vi "Answer Received.vi"(8 "error in (no error)":errorcluster, 9 "Correct?":bool, 10 "Contestant":i32, 11 "Controller in":refnum<class "Controller.lvclass">) -> (0 "error out":errorcluster, 3 "Controller out":refnum<class "Controller.lvclass">)   [LabVIEW 2024, in "Controller.lvlib" / "Controller.lvclass"]
uses:
  Controller.lvclass
  C:/Program Files/National Instruments/LabVIEW 2024/vi.lib/ActorFramework/Actor/Actor.lvclass
  Controller.lvclass/Controller.ctl
  <vilib>/ActorFramework/Message Enqueuer/Message Enqueuer.lvclass/Message Enqueuer.ctl
  Contestant/Contestant Messages/Decrement Score Msg/Decrement Score Msg.lvclass/Decrement Score Msg.ctl
  <vilib>/ActorFramework/Actor/Actor.lvclass/Actor.ctl
  Controller Messages/Update Player Who Answered Correctly Last Msg/Update Player Who Answered Correctly Last Msg.lvclass/Update Player Who Answered Correctly Last Msg.ctl
  Contestant/Contestant Messages/Increment Score Msg/Increment Score Msg.lvclass/Increment Score Msg.ctl
  <vilib>/ActorFramework/Message Enqueuer/Enqueue.vi
  <vilib>/ActorFramework/Message Enqueuer/Init from Existing Queue.vi
  Timer/Timer Messages/Stop Timer Msg/Stop Timer Msg.lvclass
  C:/Program Files/National Instruments/LabVIEW 2024/vi.lib/ActorFramework/Message/Message.lvclass
  Contestant/Contestant Messages/Decrement Score Msg/Decrement Score Msg.lvclass
  Contestant/Contestant Messages/Light to Red Msg/Light to Red Msg.lvclass
  Controller Messages/Update Player Who Answered Correctly Last Msg/Update Player Who Answered Correctly Last Msg.lvclass
  Contestant/Contestant Messages/Increment Score Msg/Increment Score Msg.lvclass
  <vilib>/ActorFramework/Message Priority Queue/Priority Enqueue.vi
  <vilib>/ActorFramework/Message Enqueuer/Message Enqueuer.lvclass
  <vilib>/ActorFramework/Actor/Actor.lvclass
  C:/Users/ekerry/Documents/challenge-of-champions/Controller/Controller/Controller.lvclass
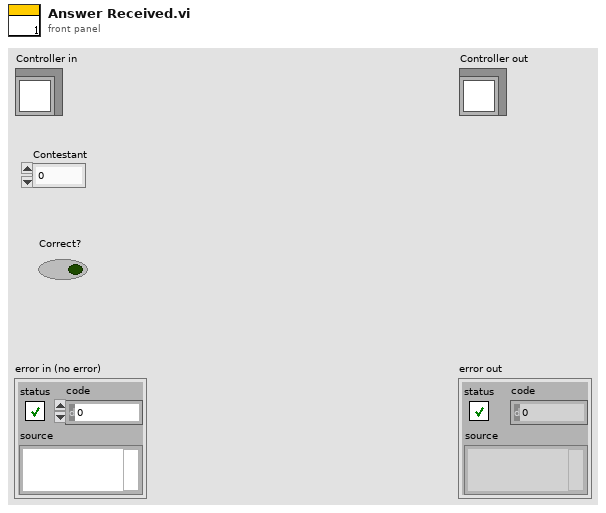
[diagram p1: front panel]
types:
  T1 = map{i32, refnum<class "Message Enqueuer.lvclass">}
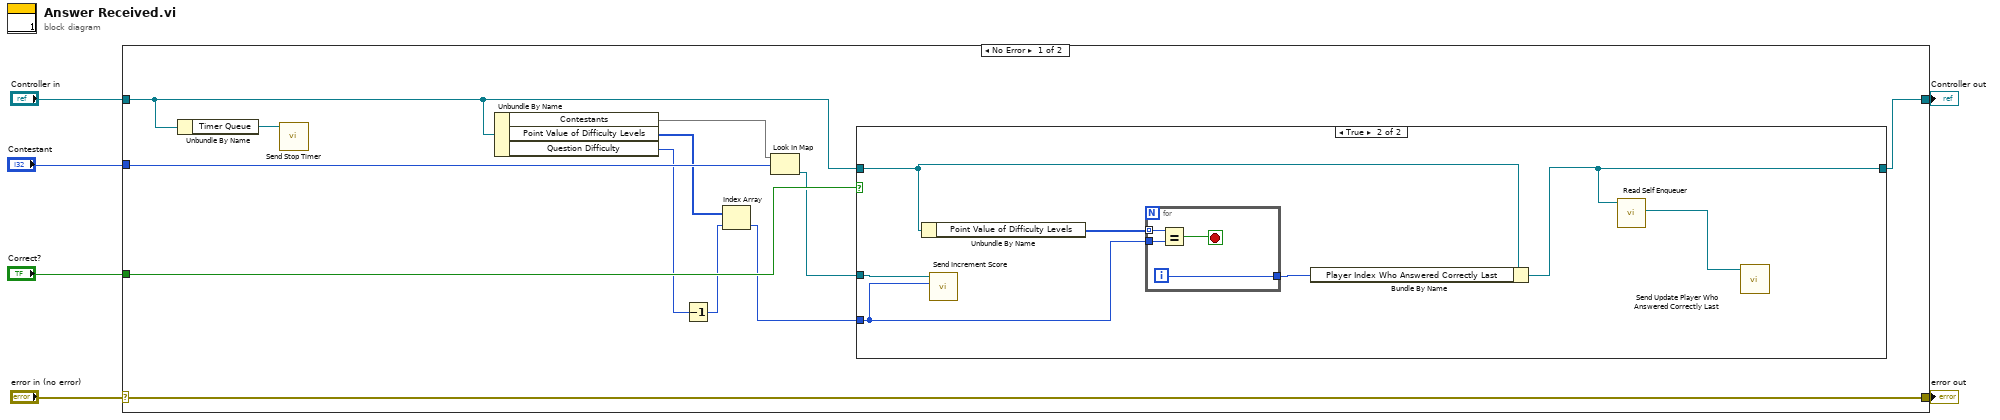
[diagram p0: block diagram]
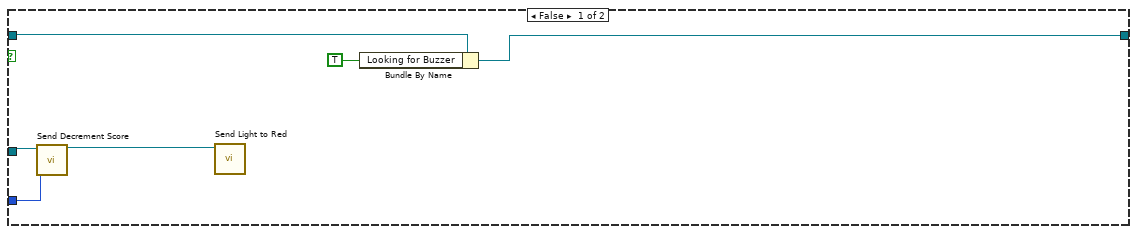
[diagram p2: hidden frame]
diagram:
  n1 = case shown="No Error" "error in (no error)" {
    selector: "error in (no error)" -> [w18 w37]
    tunnel: [w18 w37] -> w5
    tunnel: [w9 w36] -> w3
    tunnel: "Controller in" -> [w8 w36]
    tunnel: "Contestant" -> [w16 _]
    tunnel: "Correct?" -> [w15 _]
    frame No Error {
      n2 = Unbundle By Name(w8) -> ("Timer Queue"=w7:refnum<class "Message Enqueuer.lvclass">)
      n3 = call "Send Stop Timer.vi"("Message Enqueuer"=w7) -> ()  [unwired: 9 in, 2 out]
      n4 = Unbundle By Name(w8) -> ("Contestants"=w17:T1, "Point Value of Difficulty Levels"=w13:i32[], "Question Difficulty"=w11:i32)
      n5 = Decrement(x=w11) -> (x-1=w10:i32)
      n6 = Index Array(array=w13, index=w10) -> (element=w12:i32)
      n7 = Look In Map(map=w17, key=w16) -> (value=w14:refnum<class "Message Enqueuer.lvclass">)  [unwired: 1 in, 1 out]
      n8 = case shown="True" w15 {
        tunnel: w14 -> [w21 w31]
        tunnel: w12 -> [w20 w28]
        tunnel: w8 -> [w24 w27]
        tunnel: [w23 w26] -> w9
        frame False {
          n9 = call "Send Decrement Score.vi"("Points Lost"=w20, "Message Enqueuer"=w21) -> ("Message Enqueuer out"=w19:refnum<class "Message Enqueuer.lvclass">)  [unwired: 8 in, 1 out]
          n10 = call "Send Light to Red.vi"("Message Enqueuer"=w19) -> ()  [unwired: 9 in, 2 out]
          n11 = Bundle By Name(cluster=w24, "Looking for Buzzer"=TRUE) -> (w23:refnum<class "Controller.lvclass">)
        }
        frame True {
          n12 = Unbundle By Name(w27) -> ("Point Value of Difficulty Levels"=w29:i32[])
          n13 = call "Send Increment Score.vi"("Points Awarded"=w28, "Message Enqueuer"=w31) -> ()  [unwired: 8 in, 2 out]
          n14 = for {
            tunnel: w29 -> [w35] mode=indexing
            tunnel: w28 -> [w34]
            tunnel: [w33] -> w25
            i -> [w33]
            stop <- w32 stop-if-true
            n15 = Equal?(x=w35, y=w34) -> (x = y?=w32:bool)
          }
          n16 = Bundle By Name(cluster=w27, "Player Index Who Answered Correctly Last"=w25) -> (w26:refnum<class "Controller.lvclass">)
          n17 = call <vilib>:"Read Self Enqueuer.vi"("Actor"=w26) -> ("Self Enqueuer"=w30:refnum<class "Message Enqueuer.lvclass">)  [unwired: 10 in]
          n18 = call "Send Update Player Who Answered Correctly Last.vi"("Message Enqueuer"=w30) -> ()  [unwired: 9 in, 2 out]
        }
      }
    }
    frame Error {
    }
  }
  "error out" <- w5
  "Controller out" <- w3
